vi "CMD_Drive.vi"(1 "Line":string) -> (0 "Done":bool)   [LabVIEW 2014]
uses:
  Robot Global Data.vi
  <vilib>/addons/control/pid/pid.llb/PID (DBL).vi
  <vilib>/addons/control/pid/NI_PID_pid.lvlib
  navX-MXP Library/navX-MXP IMU.lvlib
panel:
  in  "Parameters":i32[](array[numeric])=[1, 3, 1, 3, 1]
  in  "Subcommands":string[](array[string])=["at", "at", "for", "to", "until"]
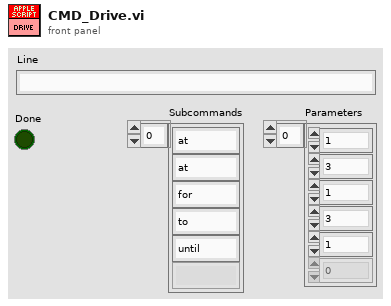
[diagram p1: front panel]
types:
  T1 = cluster{"proportional gain (Kc)":dbl, "integral time (Ti, min)":dbl, "derivative time (Td, min)":dbl}
  T2 = typedef "navX-MXP IMU.lvlib/navX SPI DevRef.ctl" = cluster{"SPIDevRef":T3, "Board Information":T6, "Status":T7, "Offsets":cluster{"Yaw":dbl, "Quat W":dbl, "Quat X":dbl, "Quat Y":dbl, "Quat Z":dbl}, "Update Rate (4Hz-60Hz)":u8, "refnum name":string, "error":errorcluster}
  T3 = typedef "WPI_SPIDevRef.ctl" = cluster{"DevStatus":errorcluster, "Handle":i32, "Controller":T4, "SPI Bus":T5}
  T4 = typedef "FPGA_TypedefDigitalModule.ctl" = enum16{"Controller 1"}
  T5 = typedef "spi_bus.ctl" = enum16{"SPI On-Board, CS0", "SPI On-Board, CS1", "SPI On-Board, CS2", "SPI On-Board, CS3", "SPI MXP", "Invalid"}
  T6 = typedef "navX-MXP IMU.lvlib/navX Board Information.ctl" = cluster{"WhoAmI (50 | 0x32)":u8, "Board Revision":u8, "Firmware Major Version":u8, "Firmware Minor Version":u8}
  T7 = typedef "navX-MXP IMU.lvlib/navX Status Data.ctl" = cluster{"Update Rate Hz":u8, "Accelerometer Full-Scale Range":u8, "Gyro Full-Scale Range":u16, "NAVX_OP_STATUS":T8, "NAVX_CAL_STATUS":T9, "NAVX_SELFTEST_STATUS":u8, "NAVX_SENSOR_STATUS":T10}
  T8 = typedef "navX-MXP IMU.lvlib/navX NAVX_OP_STATUS.ctl" = u8
  T9 = typedef "navX-MXP IMU.lvlib/navX NAVX_CAL_STATUS.ctl" = u8
  T10 = typedef "navX-MXP IMU.lvlib/navX NAVX_SENSOR_STATUS.ctl" = cluster{"MOVING":bool, "YAW_STABLE":bool, "MAG_DISTURBANCE":bool, "ALTITUDE_VALID":bool, "SEALEVEL_PRESS_SET":bool, "FUSED_HEADING_VALID":bool}
  T11 = typedef "navX-MXP IMU.lvlib/navX YPRH Data.ctl" = cluster{"Yaw":dbl, "Pitch":dbl, "Roll":dbl, "Heading":dbl}
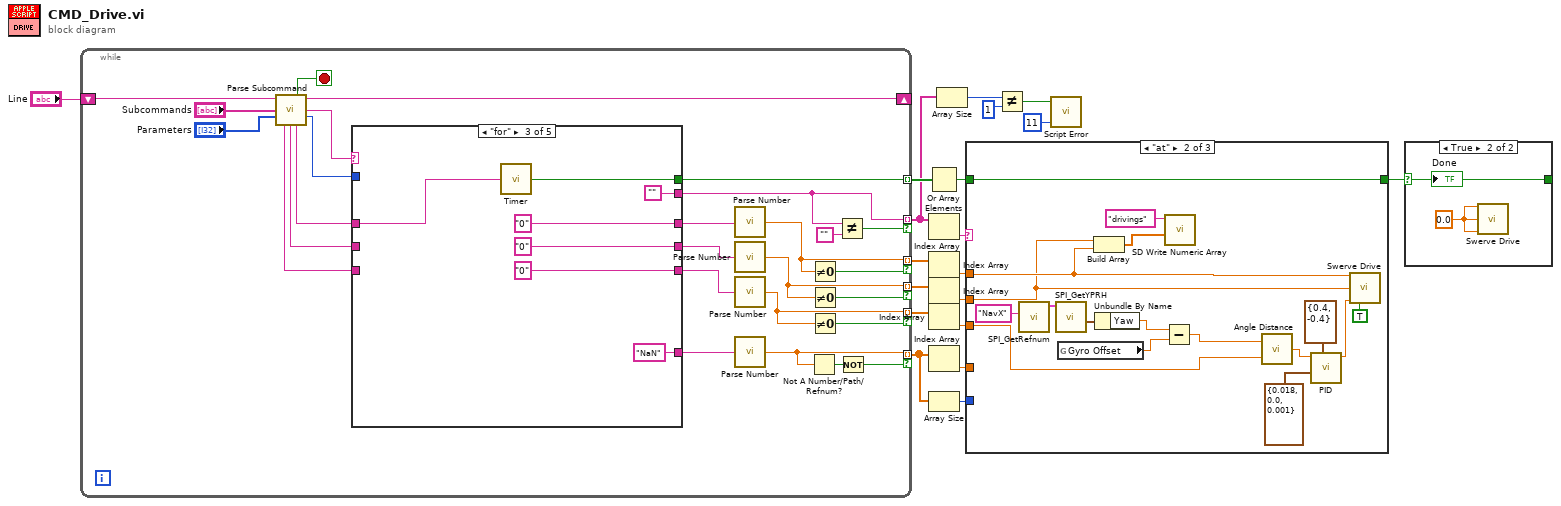
[diagram p0: block diagram]
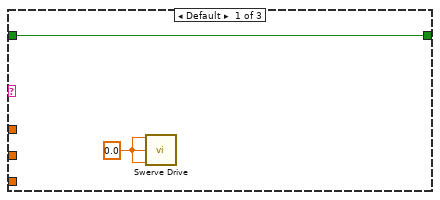
[diagram p3: hidden frame]
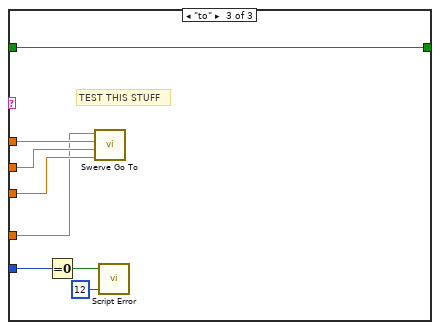
[diagram p4: hidden frame]
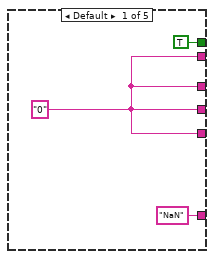
[diagram p5: hidden frame]
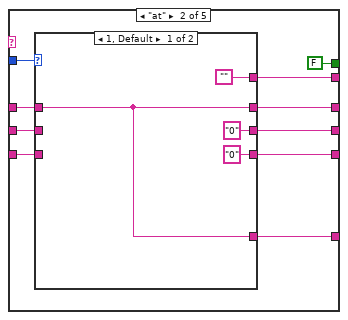
[diagram p6: hidden frame]
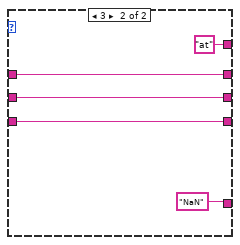
[diagram p7: hidden frame]
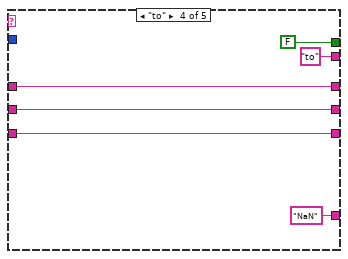
[diagram p8: hidden frame]
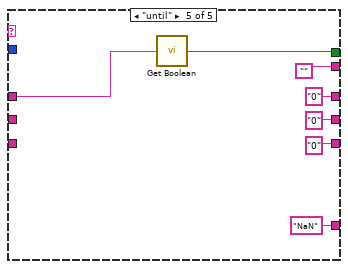
[diagram p9: hidden frame]
diagram:
  n1 = while {
    shift-right: [w44] -> _
    shift-left: "Line" -> [w47]
    tunnel: [w21] -> w5 mode=indexing
    tunnel: [w33] -> w17 mode=indexing if=w27
    tunnel: [w32] -> w15 mode=indexing if=w25
    tunnel: [w29] -> w13 mode=indexing if=w26
    tunnel: [w24] -> w3 mode=indexing if=w22
    tunnel: [w35] -> w4 mode=indexing if=w36
    stop <- w43 stop-if-true
    n2 = call "Parse Subcommand.vi"("Text In"=w47, "Subcommands"="Subcommands", "Parameters"="Parameters") -> ("Done"=w43:bool, "Text Out"=w44:string, "Subcommand"=w42:string, "# of Parameters"=w41:i32, "Parameter 3"=w39:string, "Parameter 2"=w38:string, "Parameter 1"=w40:string)  [unwired: 6 in]
    n3 = case shown="\"for\"" w42 {
      tunnel: w41 -> [_ w60 _ _ _]
      tunnel: w40 -> [_ w59 w70 w82 w84]
      tunnel: w38 -> [_ w58 _ w81 _]
      tunnel: w39 -> [_ w57 _ w80 _]
      tunnel: [w49 w56 "0" ("Parameter 1") w82 "0" ("Parameter 1")] -> w34
      tunnel: [w49 w55 "0" ("Parameter 2") w81 "0" ("Parameter 1")] -> w31
      tunnel: [w49 w54 "0" ("Parameter 3") w80 "0" ("Parameter 1")] -> w30
      tunnel: [TRUE ("Value") FALSE ("Running") w71 FALSE w83] -> w21
      tunnel: [w49 w51 "" "to" ("format string") ""] -> w35
      tunnel: ["NaN" ("Parameter 1") w53 "NaN" ("Parameter 3") "NaN" ("Parameter 3") "NaN" ("Parameter 1")] -> w28
      frame Default {
        w49 = "0" ("format string")
      }
      frame "at" {
        n4 = case shown="1, Default" w60 {
          tunnel: w59 -> [w62 w69]
          tunnel: w58 -> [_ w68]
          tunnel: w57 -> [_ w65]
          tunnel: [w62 w69] -> w56
          tunnel: ["0" ("Parameter 2") w68] -> w55
          tunnel: ["0" ("Parameter 3") w65] -> w54
          tunnel: [w62 "NaN" ("Parameter 3")] -> w53
          tunnel: ["" "at"] -> w51
          frame 1, Default {
          }
          frame 3 {
          }
        }
      }
      frame "for" {
        n5 = call "Timer.vi"("Seconds (string)"=w70) -> ("Done"=w71:bool)
      }
      frame "to" {
      }
      frame "until" {
        n6 = call "Get Boolean.vi"("Name"=w84) -> ("Value"=w83:bool)
      }
    }
    n7 = call "Parse Number.vi"("String"=w34) -> ("Number"=w33:dbl)
    n8 = call "Parse Number.vi"("String"=w31) -> ("Number"=w32:dbl)
    n9 = call "Parse Number.vi"("String"=w30) -> ("Number"=w29:dbl)
    n10 = call "Parse Number.vi"("String"=w28) -> ("Number"=w24:dbl)
    n11 = Not A Number/Path/Refnum?(number/path/refnum=w24) -> (NaN/Path/Refnum?=w23:bool)
    n12 = Not Equal To 0?(x=w33) -> (x != 0?=w27:bool)
    n13 = Not Equal To 0?(x=w32) -> (x != 0?=w25:bool)
    n14 = Not Equal To 0?(x=w29) -> (x != 0?=w26:bool)
    n15 = Not Equal?(x=w35, y="") -> (x != y?=w36:bool)
    n16 = Not(x=w23) -> (.not. x?=w22:bool)
  }
  n17 = Or Array Elements(Boolean array=w5) -> (logical OR=w1:bool)
  n18 = Index Array(array=w4) -> (element=w10:string)  [unwired: 1 in]
  n19 = Index Array(array=w17) -> (element=w16:dbl)  [unwired: 1 in]
  n20 = Index Array(array=w15) -> (element=w14:dbl)  [unwired: 1 in]
  n21 = Index Array(array=w13) -> (element=w12:dbl)  [unwired: 1 in]
  n22 = Index Array(array=w3) -> (element=w11:dbl)  [unwired: 1 in]
  n23 = Array Size(array=w3) -> (size(s)=w2:i32)
  n24 = Array Size(array=w4) -> (size(s)=w8:i32)
  n25 = case shown="\"at\"" w10 {
    tunnel: w16 -> [_ w102 w115]
    tunnel: w1 -> [w91 w108 w116]
    tunnel: [w91 w108 w116] -> w18
    tunnel: w14 -> [_ w101 w114]
    tunnel: w12 -> [_ w92 w113]
    tunnel: w11 -> [_ _ w112]
    tunnel: w2 -> [_ _ w110]
    frame Default {
      w90 = 0.0 ("X")
      n26 = call "Swerve Drive.vi"("X"=w90, "Y"=w90, "Z"=w90) -> ()  [unwired: 13 in]
    }
    frame "at" {
      n27 = call "SPI_GetRefnum.vi"("refnum name"="NavX") -> ("navX DevRef"=w97:T2)  [unwired: 9 in, 1 out]
      n28 = call "SPI_GetYPRH.vi"("navX DevRef"=w97) -> ("YPRH"=w96:T11)  [unwired: 8 in, 2 out]
      n29 = global read "Robot Global Data.vi" "Gyro Offset"() -> (w95:dbl)
      n30 = Build Array(w101, w102) -> (w100:dbl[])
      n31 = Unbundle By Name(w96) -> ("Yaw"=w94:dbl)
      n32 = Subtract(x=w94, y=w95) -> (x-y=w93:dbl)
      n33 = call <vilib>:"SD Write Numeric Array.vi"("Numeric Array"=w100, "Name"="drivings") -> ()  [unwired: 8 in, 2 out]
      n34 = call "Angle Distance.vi"("target angle"=w92, "current angle"=w93) -> ("distance"=w99:dbl)
      n35 = call-poly <vilib>:"PID.vi"("output range"=cluster{"output high":dbl, "output low":dbl} {"output high"=0.4, "output low"=-0.4}, "PID gains"=T1 {"proportional gain (Kc)"=0.018, "integral time (Ti, min)"=0.0, "derivative time (Td, min)"=0.001}, "setpoint"=w99) -> ("output"=w104:dbl)  [unwired: 7 in, 1 out]
      n36 = call "Swerve Drive.vi"("X"=w102, "Y"=w101, "Z"=w104, "Auto Controls"=TRUE) -> ()  [unwired: 12 in]
    }
    frame "to" {
      # "TEST THIS STUFF"
      n37 = Equal To 0?(x=w110) -> (x = 0?=w109:bool)
      n38 = call "Swerve Go To.vi"("Max Speed"=w112, "Target X"=w115, "Target Y"=w114, "Target Angle"=w113) -> ()  [unwired: 3 in, 1 out]
      n39 = call "Script Error.vi"("Error?"=w109, "Error Code"=12) -> ()  [unwired: 3 in, 1 out]
    }
  }
  n40 = Not Equal?(x=w8, y=1) -> (x != y?=w6:bool)
  n41 = call "Script Error.vi"("Error?"=w6, "Error Code"=11) -> ()  [unwired: 3 in, 1 out]
  n42 = case shown="True" w18 {
    selector: w18 -> [w117 w119]
    tunnel: [w117 w119] -> w19
    frame False {
    }
    frame True {
      w118 = 0.0 ("X")
      n43 = call "Swerve Drive.vi"("X"=w118, "Y"=w118, "Z"=w118) -> ()  [unwired: 13 in]
    }
  }
  "Done" <- w19
